vi "End.vi"(8 "error in (no error)":errorcluster, 11 "AutoExp in":refnum<class "AutoExp.lvclass">) -> (0 "error out":errorcluster, 3 "AutoExp out":refnum<class "AutoExp.lvclass">)   [LabVIEW 2018, in "AutoExp.lvclass"]
uses:
  AutoExp.lvclass
  AutoExp.lvclass/AutoExp.ctl
  Channel/Channel.lvclass
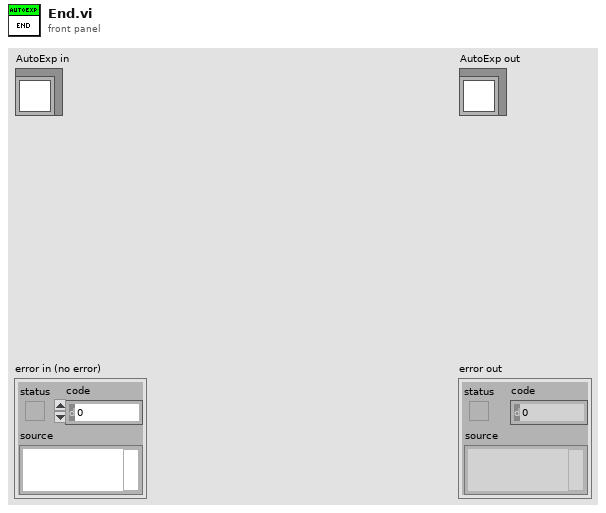
[diagram p1: front panel]
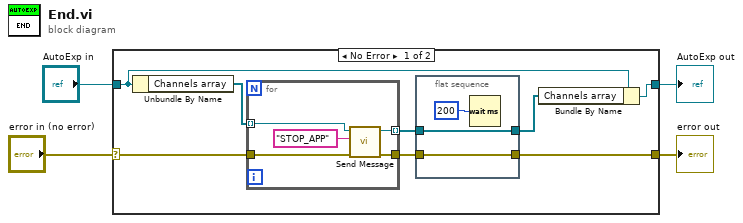
[diagram p0: block diagram]
diagram:
  n1 = case shown="No Error" "error in (no error)" {
    selector: "error in (no error)" -> [w11 w22]
    tunnel: [w7 w22] -> w3
    tunnel: [w9 w21] -> w1
    tunnel: "AutoExp in" -> [w10 w21]
    frame No Error {
      n2 = Unbundle By Name(w10) -> ("Channels array"=w12:refnum<class "Channel.lvclass">[])
      n3 = for {
        tunnel: w12 -> [w20] mode=indexing
        tunnel: w11 -> [w19]
        tunnel: [w17] -> w8
        tunnel: [w16] -> w6 mode=indexing
        n4 = call "Send Message.vi"("error in (no error)"=w19, "message"="STOP_APP", "Channel in"=w20) -> ("error out"=w17:errorcluster, "Channel out"=w16:refnum<class "Channel.lvclass">)  [unwired: 7 in]
      }
      n5 = flat-sequence {
        tunnel: [w15] -> w7
        tunnel: w8 -> [w15]
        tunnel: w6 -> [w13]
        tunnel: [w13] -> w5
        frame #0 {
          n6 = Wait (ms)(milliseconds to wait=u32 200) -> ()  [unwired: 1 out]
        }
      }
      n7 = Bundle By Name(cluster=w10, "Channels array"=w5) -> (w9:refnum<class "AutoExp.lvclass">)
    }
    frame Error {
    }
  }
  "error out" <- w3
  "AutoExp out" <- w1
